vi "ExpandLinkAndRedirectGraph.vi"(8 "error in (no error)":errorcluster, 10 "GraphNode in":refnum<data-value>, 11 "Graph in":refnum<class "Graph.lvclass">) -> (0 "error out":errorcluster, 1 "ExpandedNodes":refnum<data-value>[](array[refnum]), 2 "GraphNode out":refnum<data-value>, 3 "Graph out":refnum<class "Graph.lvclass">)   [LabVIEW 2010, in "Graph.lvclass"]
doc: "Expands Nodes to search through in the graph. Expanded nodes are linked to the graph, and depending on their evaluation can have their tracer changed."
uses:
  Graph.lvclass
  GraphNode/GraphNode.lvclass
  Graph.lvclass/Graph.ctl
  LinkedList/LinkedList.lvclass
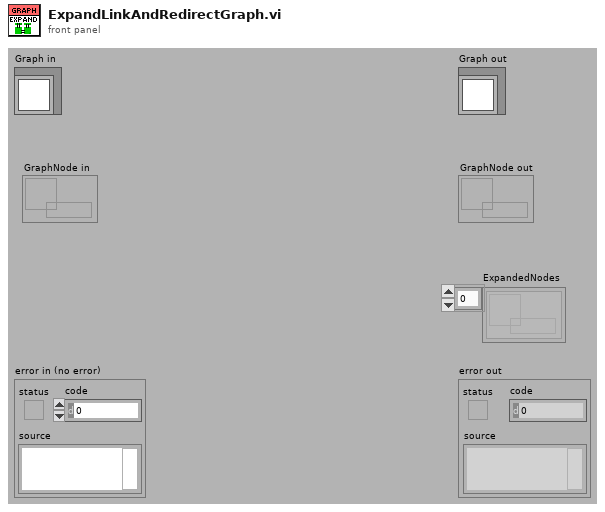
[diagram p1: front panel]
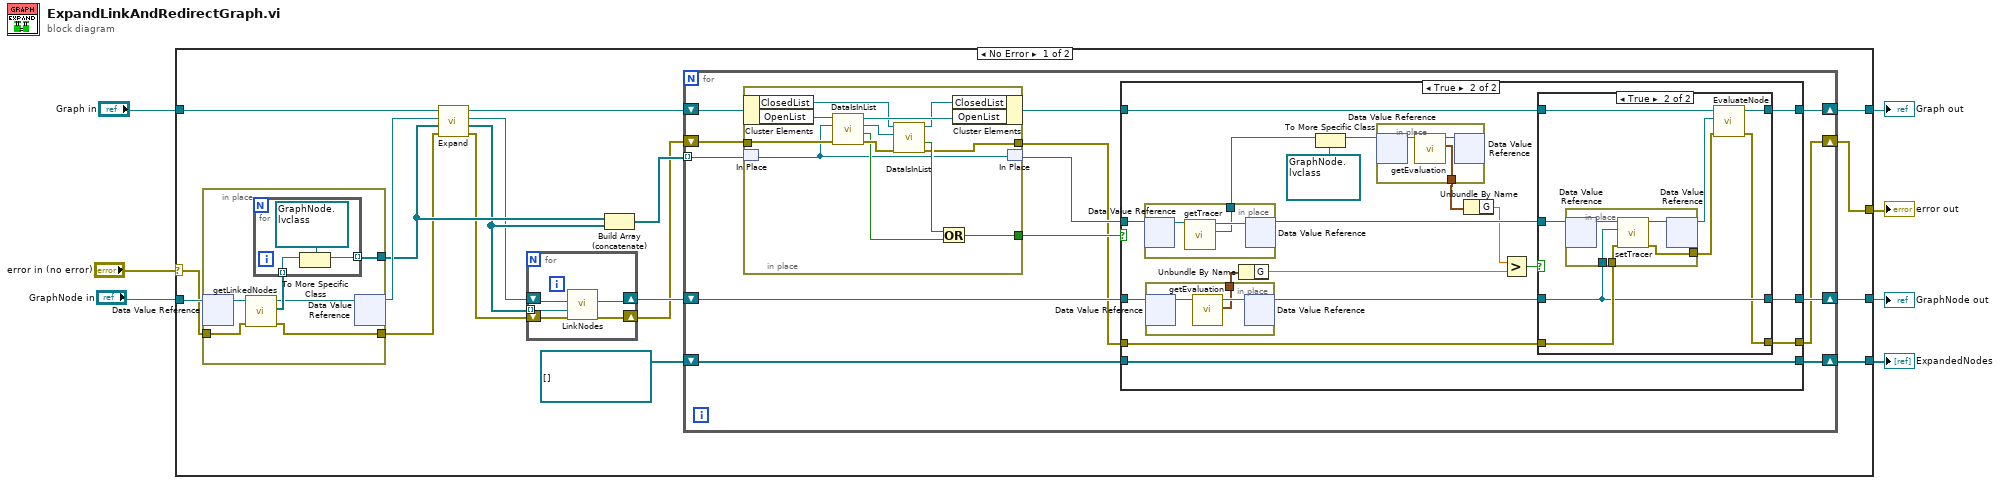
[diagram p0: block diagram]
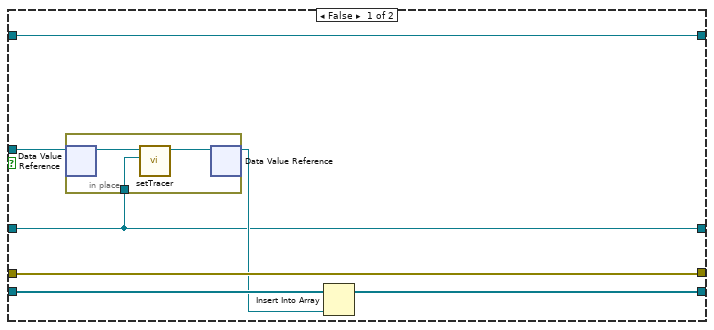
[diagram p2: hidden frame]
diagram:
  n1 = case shown="No Error" "error in (no error)" {
    selector: "error in (no error)" -> [w24 w120]
    tunnel: [w19 w120] -> w2
    tunnel: [w22 w119] -> w6
    tunnel: "Graph in" -> [w18 w119]
    tunnel: "GraphNode in" -> [w25 w118]
    tunnel: [w21 _] -> w1
    tunnel: [w20 w118] -> w3
    frame No Error {
      n2 = in-place {
        in-place-border: w24 -> [w113]
        in-place-border: [w110] -> w10
        in-place-border: [w109] -> w15
        n3 = in-place-dvr #1(w25) -> (w114:refnum<class "GraphNode.lvclass">)  [unwired: 1 out]
        n4 = call "getLinkedNodes.vi"("error in (no error)"=w113, "GraphNode in"=w114) -> ("error out"=w110:errorcluster, "LinkedNodes"=w112:refnum<data-value>[], "GraphNode out"=w111:refnum<class "GraphNode.lvclass">)  [unwired: 7 in]
        n5 = for {
          tunnel: w112 -> [w117] mode=indexing
          tunnel: [w115] -> w109 mode=indexing
          n6 = To More Specific Class(target class=refnum<data-value> refnum ("GraphNode out 2"), reference=w117) -> (specific class reference=w115:refnum<data-value>)  [unwired: 1 in, 1 out]
        }
        n7 = in-place-dvr #1(w111) -> (w16:refnum<data-value>)  [unwired: 1 out]
      }
      n8 = call-dynamic "Expand.vi"("error in (no error)"=w10, "CurrentLinkedNodes"=w15, "NodeToExpand in"=w16, "Graph in"=w18) -> ("error out"=w9:errorcluster, "NodesToLinkAndExpand"=w13:refnum<data-value>[], "NodeToExpand out"=w12:refnum<data-value>, "Graph out"=w17:refnum<class "Graph.lvclass">)  [unwired: 4 in]
      n9 = for {
        tunnel: w13 -> [w30] mode=indexing
        shift-right: [w28] -> w11
        shift-left: w12 -> [w29]
        shift-right: [w26] -> w8
        shift-left: w9 -> [w27]
        n10 = call "LinkNodes.vi"("error in (no error)"=w27, "GraphNode2 in"=w30, "GraphNode1 in"=w29) -> ("error out"=w26:errorcluster, "GraphNode1 out"=w28:refnum<data-value>)  [unwired: 6 in, 1 out]
      }
      n11 = Build Array (concatenate)(w15, w13) -> (w14:refnum<data-value>[])
      n12 = for {
        tunnel: w14 -> [w31] mode=indexing
        shift-right: [w36] -> w22
        shift-left: w17 -> [w43]
        shift-right: [w37] -> w21
        shift-left: refnum<data-value>[] [] -> [w38]
        shift-right: [w33] -> w20
        shift-left: w11 -> [w35]
        shift-right: [w32] -> w19
        shift-left: w8 -> [w42]
        n13 = in-place {
          in-place-border: w42 -> [w106]
          in-place-border: [w98] -> w41
          in-place-border: [w97] -> w34
          n14 = in-place-cluster #2(w43) -> ("ClosedList"=w105:refnum<class "BasicSortedList.lvclass">, "OpenList"=w108:refnum<class "BasicSortedList.lvclass">)
          n15 = in-place-match #3(w31) -> (w99:refnum<data-value>)
          n16 = call "DataIsInList.vi"("error in (no error)"=w106, "LLNode in"=w99, "LinkedList in"=w108) -> ("error out"=w102:errorcluster, "inList"=w100:bool, "LLNode out"=w103:refnum<data-value>, "LinkedList out"=w107:refnum<class "BasicSortedList.lvclass">)  [unwired: 4 in, 1 out]
          n17 = call "DataIsInList.vi"("error in (no error)"=w102, "LLNode in"=w103, "LinkedList in"=w105) -> ("error out"=w97:errorcluster, "inList"=w101:bool, "LinkedList out"=w104:refnum<class "BasicSortedList.lvclass">)  [unwired: 4 in, 2 out]
          n18 = Or(x=w101, y=w100) -> (x .or. y?=w98:bool)
          n19 = in-place-cluster #2("ClosedList"=w104, "OpenList"=w107) -> (w40:refnum<class "Graph.lvclass">)
          n20 = in-place-match #3(w99) -> (w39:refnum<data-value>)
        }
        n21 = case shown="True" w41 {
          tunnel: w40 -> [w48 w60]
          tunnel: w39 -> [w46 w69]
          tunnel: w38 -> [w50 w71]
          tunnel: [w49 w71] -> w37
          tunnel: [w48 w59] -> w36
          tunnel: w35 -> [w44 w70]
          tunnel: w34 -> [w47 w62]
          tunnel: [w44 w61] -> w33
          tunnel: [w47 w58] -> w32
          frame False {
            n22 = in-place {
              in-place-border: w44 -> [w51]
              n23 = in-place-dvr #4(w46) -> (w53:refnum<class "GraphNode.lvclass">)  [unwired: 1 out]
              n24 = call "setTracer.vi"("tracer"=w51, "GraphNode in"=w53) -> ("GraphNode out"=w52:refnum<class "GraphNode.lvclass">)  [unwired: 8 in, 1 out]
              n25 = in-place-dvr #4(w52) -> (w45:refnum<data-value>)  [unwired: 1 out]
            }
            n26 = Insert Into Array(array=w50, new element=w45) -> (w49:refnum<data-value>[])  [unwired: 1 in]
          }
          frame True {
            n27 = in-place {
              in-place-border: [w91] -> w68
              n28 = in-place-dvr #5(w69) -> (w93:refnum<class "GraphNode.lvclass">)  [unwired: 1 out]
              n29 = call "getTracer.vi"("GraphNode in"=w93) -> ("tracer"=w91:refnum<data-value>, "GraphNode out"=w92:refnum<class "GraphNode.lvclass">)  [unwired: 8 in, 1 out]
              n30 = in-place-dvr #5(w92) -> (w64:refnum<data-value>)  [unwired: 1 out]
            }
            n31 = in-place {
              in-place-border: [w94] -> w57
              n32 = in-place-dvr #6(w70) -> (w96:refnum<class "GraphNode.lvclass">)  [unwired: 1 out]
              n33 = call "getEvaluation.vi"("GraphNode in"=w96) -> ("Evaluation"=w94:cluster{"F":dbl, "G":dbl, "H":dbl}, "GraphNode out"=w95:refnum<class "GraphNode.lvclass">)  [unwired: 8 in, 1 out]
              n34 = in-place-dvr #6(w95) -> (w63:refnum<data-value>)  [unwired: 1 out]
            }
            n35 = Unbundle By Name(w57) -> ("G"=w56:dbl)
            n36 = To More Specific Class(target class=refnum<data-value> refnum ("GraphNode out 2"), reference=w68) -> (specific class reference=w66:refnum<data-value>)  [unwired: 1 in, 1 out]
            n37 = in-place {
              in-place-border: [w88] -> w55
              n38 = in-place-dvr #7(w66) -> (w90:refnum<class "GraphNode.lvclass">)  [unwired: 1 out]
              n39 = call "getEvaluation.vi"("GraphNode in"=w90) -> ("Evaluation"=w88:cluster{"F":dbl, "G":dbl, "H":dbl}, "GraphNode out"=w89:refnum<class "GraphNode.lvclass">)  [unwired: 8 in, 1 out]
              n40 = in-place-dvr #7(w89) -> ()  [unwired: 2 out]
            }
            n41 = Unbundle By Name(w55) -> ("G"=w54:dbl)
            n42 = Greater?(x=w54, y=w56) -> (0:w65:bool)
            n43 = case shown="True" w65 {
              tunnel: w64 -> [_ w82]
              tunnel: w63 -> [w74 w80]
              tunnel: w62 -> [w72 w81]
              tunnel: [w74 w80] -> w61
              tunnel: w60 -> [w73 w79]
              tunnel: [w73 w77] -> w59
              tunnel: [w72 w75] -> w58
              frame False {
              }
              frame True {
                n44 = in-place {
                  in-place-border: w80 -> [w86]
                  in-place-border: w81 -> [w85]
                  in-place-border: [w83] -> w76
                  n45 = in-place-dvr #8(w82) -> (w87:refnum<class "GraphNode.lvclass">)  [unwired: 1 out]
                  n46 = call "setTracer.vi"("error in (no error)"=w85, "tracer"=w86, "GraphNode in"=w87) -> ("error out"=w83:errorcluster, "GraphNode out"=w84:refnum<class "GraphNode.lvclass">)  [unwired: 7 in]
                  n47 = in-place-dvr #8(w84) -> (w78:refnum<data-value>)  [unwired: 1 out]
                }
                n48 = call "EvaluateNode.vi"("error in (no error)"=w76, "ToEvaluate in"=w78, "Graph in"=w79) -> ("error out"=w75:errorcluster, "Graph out"=w77:refnum<class "Graph.lvclass">)  [unwired: 6 in, 1 out]
              }
            }
          }
        }
      }
    }
    frame Error {
    }
  }
  "error out" <- w2
  "Graph out" <- w6
  "GraphNode out" <- w3
  "ExpandedNodes" <- w1
